vi "testXcontrol1.vi"() -> ()   [LabVIEW 2018]
uses:
  XControl 1.xctl
  <vilib>/Utility/miscctls.llb/LVPointDoubleTypeDef.ctl
  <vilib>/Analysis/baseanly.llb/Real Outer Product.vi
  <vilib>/Analysis/Matrix/Numeric/Conversions/Matrix To Array - RM.vi
  <vilib>/Analysis/NI_AALBase.lvlib
  <vilib>/Analysis/Matrix/NI_Matrix.lvlib
panel:
  out "XControl 1":T2(xcontrol)
  in  "Stop Button":bool
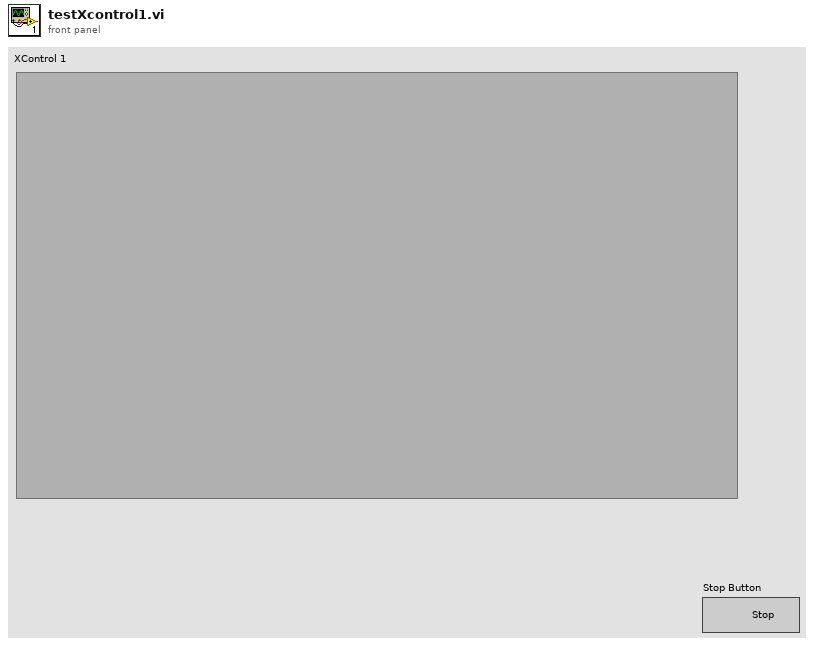
[diagram p1: front panel]
types:
  T1 = typedef "LVPointDoubleTypeDef.ctl" = cluster{"X":dbl, "Y":dbl}
  T2 = cluster{"Cluster":cluster{"2^n : x":i8, "2^n : y":i8, "lower left box Position":T1}, "Array":dbl[][]}
  T3 = typedef "NI_Matrix.lvlib/RealMatrix.ctl" = dbl[][]
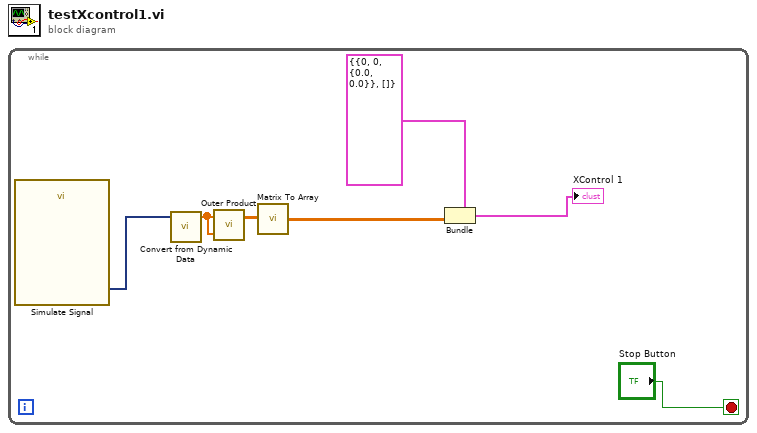
[diagram p0: block diagram]
diagram:
  n1 = while {
    stop <- "Stop Button" stop-if-true
    n2 = call "Simulate Signal"() -> ("Sine with Inverse F Noise"=w5:dynamicdata)  [unwired: 14 in, 1 out]
    n3 = call "Convert from Dynamic Data"("Dynamic Data Type"=w5) -> ("Array"=w4:dbl[])  [unwired: 3 in]
    n4 = call-poly <vilib>:"Outer Product.vi"("Y Vector"=w4, "X Vector"=w4) -> ("Outer Product"=w6:T3)  [unwired: 1 out]
    n5 = call-poly <vilib>:"Matrix To Array.vi"("Real Matrix"=w6) -> ("Real 2D Array"=w2:dbl[][])
    n6 = Bundle(cluster=T2 {"Cluster"={"2^n : x"=0, "2^n : y"=0, "lower left box Position"={"X"=0.0, "Y"=0.0}}, "Array"=[]} ("XControl 1"), "Array"=w2) -> (→"XControl 1":T2)  [unwired: 1 in]
  }
